vi "xijk_get_spectra.vi"(8 "error in":errorcluster, 10 "filepaths in":T2, 11 "spectra parameters in":T3={"Booleans"={"Notch filtering"=FALSE, "Unknown detector"=FALSE, "Dual band filters"=FALSE, "Dual emission by cubes"=FALSE, "FRET"=FALSE}, "Integers"={"Light source"=0, "Number of fluorophores"=0, "Wavelength of laser (nm) 1"=0, "Broadness of laser (nm) 1"=0.0, "Wavelength of laser (nm) 2"=0, "Broadness of laser (nm) 2"=0.0, "Template"=1}, "Doubles"={"Molar extinction 1"=1.0, "Molar extinction 2"=1.0, "Quantum efficiency 1"=1.0, "Quantum efficiency 2"=1.0}}) -> (0 "error out":errorcluster, 3 "spectra out":T1)   [LabVIEW 2010]
uses:
  Type Def/spectra_parameters.ctl
  Type Def/filepath.ctl
  Type Def/spectrum_table_control.ctl
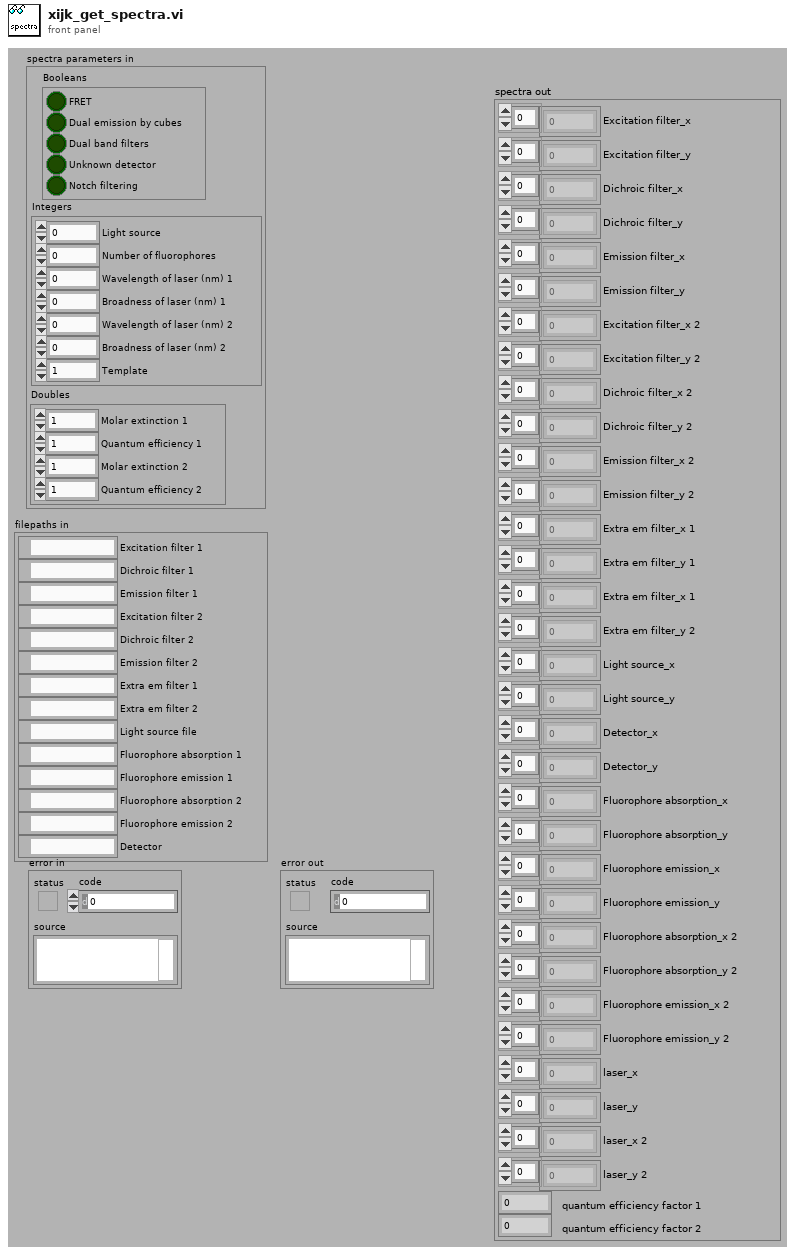
[diagram p1: front panel]
types:
  T1 = typedef "spectrum_table_control.ctl" = cluster{"Excitation filter_x":i16[], "Excitation filter_y":sgl[], "Dichroic filter_x":i16[], "Dichroic filter_y":sgl[], "Emission filter_x":i16[], "Emission filter_y":sgl[], "Excitation filter_x 2":i16[], "Excitation filter_y 2":sgl[], "Dichroic filter_x 2":i16[], "Dichroic filter_y 2":sgl[], "Emission filter_x 2":i16[], "Emission filter_y 2":sgl[], "Extra em filter_x 1":i16[], "Extra em filter_y 1":sgl[], "Extra em filter_x 1":i16[], "Extra em filter_y 2":sgl[], "Light source_x":i16[], "Light source_y":sgl[], "Detector_x":i16[], "Detector_y":sgl[], "Fluorophore absorption_x":i16[], "Fluorophore absorption_y":sgl[], "Fluorophore emission_x":i16[], "Fluorophore emission_y":sgl[], "Fluorophore absorption_x 2":i16[], "Fluorophore absorption_y 2":sgl[], "Fluorophore emission_x 2":i16[], "Fluorophore emission_y 2":sgl[], "laser_x":i16[], "laser_y":sgl[], "laser_x 2":i16[], "laser_y 2":sgl[], "quantum efficiency factor 1":sgl, "quantum efficiency factor 2":sgl}
  T2 = typedef "filepath.ctl" = cluster{"Excitation filter 1":path, "Dichroic filter 1":path, "Emission filter 1":path, "Excitation filter 2":path, "Dichroic filter 2":path, "Emission filter 2":path, "Extra em filter 1":path, "Extra em filter 2":path, "Light source file":path, "Fluorophore absorption 1":path, "Fluorophore emission 1":path, "Fluorophore absorption 2":path, "Fluorophore emission 2":path, "Detector":path}
  T3 = typedef "spectra_parameters.ctl" = cluster{"Booleans":cluster{"Notch filtering":bool, "Unknown detector":bool, "Dual band filters":bool, "Dual emission by cubes":bool, "FRET":bool}, "Integers":cluster{"Light source":u16, "Number of fluorophores":u16, "Wavelength of laser (nm) 1":u16, "Broadness of laser (nm) 1":sgl, "Wavelength of laser (nm) 2":u16, "Broadness of laser (nm) 2":sgl, "Template":u16}, "Doubles":cluster{"Molar extinction 1":sgl, "Molar extinction 2":sgl, "Quantum efficiency 1":sgl, "Quantum efficiency 2":sgl}}
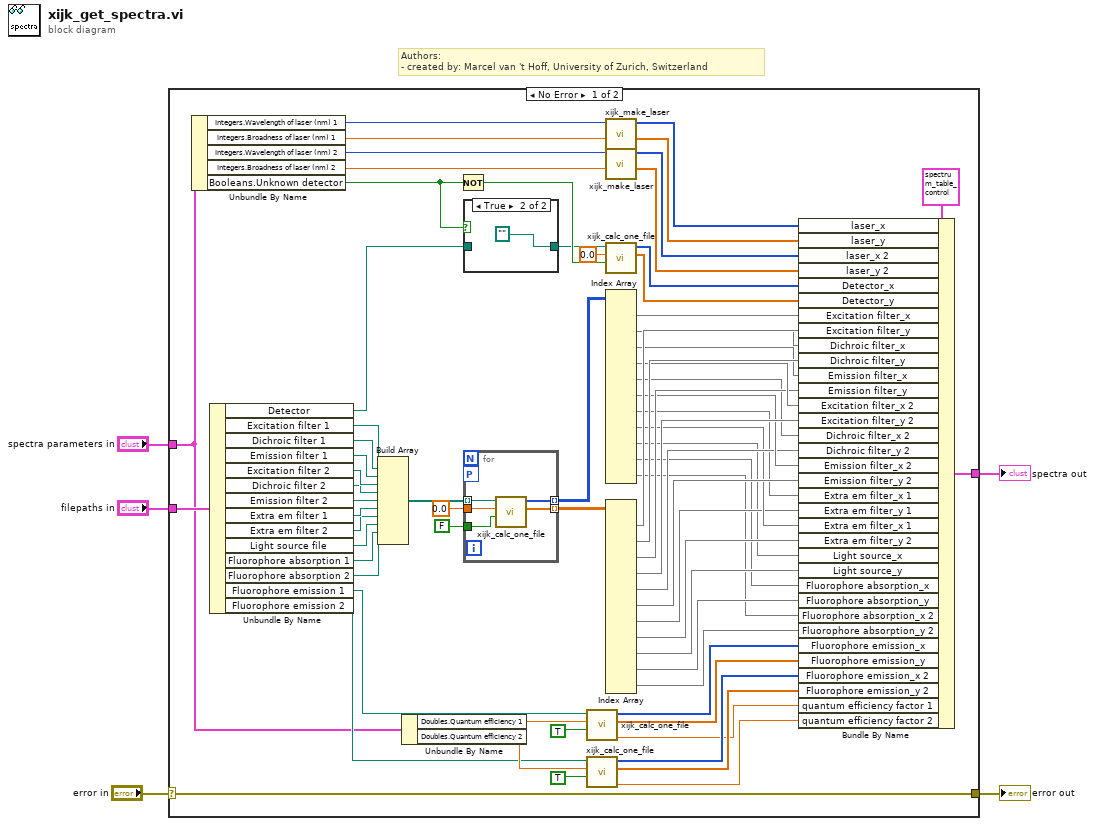
[diagram p0: block diagram]
diagram:
  # "Authors: \n- created by: Marcel van 't Hoff, University of Zurich, Switzerland"
  n1 = case shown="No Error" "error in" {
    selector: "error in" -> [w7 w83]
    tunnel: "filepaths in" -> [w75 _]
    tunnel: "spectra parameters in" -> [w50 _]
    tunnel: [w49 _] -> w3
    tunnel: [w7 w83] -> w1
    frame No Error {
      n2 = Unbundle By Name(w50) -> ("Integers.Wavelength of laser (nm) 1"=w56:u16, "Integers.Broadness of laser (nm) 1"=w55:sgl, "Integers.Wavelength of laser (nm) 2"=w54:u16, "Integers.Broadness of laser (nm) 2"=w53:sgl, "Booleans.Unknown detector"=w27:bool)
      n3 = Unbundle By Name(w75) -> ("Detector"=w28:path, "Excitation filter 1"=w74:path, "Dichroic filter 1"=w73:path, "Emission filter 1"=w72:path, "Excitation filter 2"=w71:path, "Dichroic filter 2"=w70:path, "Emission filter 2"=w69:path, "Extra em filter 1"=w68:path, "Extra em filter 2"=w64:path, "Light source file"=w67:path, "Fluorophore absorption 1"=w66:path, "Fluorophore absorption 2"=w65:path, "Fluorophore emission 1"=w52:path, "Fluorophore emission 2"=w51:path)
      n4 = Build Array(w74, w73, w72, w71, w70, w69, w68, w64, w67, w66, w65) -> (w63:path[])
      n5 = Unbundle By Name(w50) -> ("Doubles.Quantum efficiency 1"=w60:sgl, "Doubles.Quantum efficiency 2"=w57:sgl)
      n6 = Not(x=w27) -> (.not. x?=w26:bool)
      n7 = case shown="True" w27 {
        tunnel: w28 -> [w76 _]
        tunnel: [w76 path ""] -> w25
        frame False {
        }
        frame True {
        }
      }
      n8 = for {
        tunnel: w63 -> [w82] mode=indexing
        tunnel: [w81] -> w48 mode=indexing
        tunnel: [w80] -> w47 mode=indexing
        tunnel: sgl 0.0 ("quantum efficiency") -> [w79]
        tunnel: FALSE ("is_fluorophore") -> [w78]
        workers-P: _ -> [_]
        n9 = call "xijk_calc_one_file.vi"("is_fluorophore"=w78, "quantum efficiency"=w79, "input"=w82) -> ("y_out"=w80:sgl[], "x_out"=w81:i16[])  [unwired: 6 in, 1 out]
      }
      n10 = call "xijk_calc_one_file.vi"("is_fluorophore"=TRUE, "quantum efficiency"=w60, "input"=w52) -> ("quantum efficiency factor"=w9:sgl, "y_out"=w18:sgl[], "x_out"=w19:i16[])  [unwired: 6 in]
      n11 = call "xijk_calc_one_file.vi"("is_fluorophore"=TRUE, "quantum efficiency"=w57, "input"=w51) -> ("quantum efficiency factor"=w8:sgl, "y_out"=w16:sgl[], "x_out"=w17:i16[])  [unwired: 6 in]
      n12 = call "xijk_make_laser.vi"("Broadness of laser (nm)"=w55, "Wavelength of laser (nm)"=w56) -> ("laser_y"=w11:sgl[], "laser_x"=w10:i16[])  [unwired: 8 in]
      n13 = call "xijk_make_laser.vi"("Broadness of laser (nm)"=w53, "Wavelength of laser (nm)"=w54) -> ("laser_y"=w13:sgl[], "laser_x"=w12:i16[])  [unwired: 8 in]
      n14 = call "xijk_calc_one_file.vi"("is_fluorophore"=w26, "quantum efficiency"=sgl 0.0, "input"=w25) -> ("y_out"=w15:sgl[], "x_out"=w14:i16[])  [unwired: 6 in, 1 out]
      n15 = Index Array(array=w48) -> (element #1=w46:i16[], element #2=w44:i16[], element #3=w42:i16[], element #4=w41:i16[], element #5=w38:i16[], element #6=w37:i16[], element #7=w34:i16[], element #8=w33:i16[], element #9=w30:i16[], element #10=w23:i16[], element #11=w21:i16[])  [unwired: 22 in]
      n16 = Index Array(array=w47) -> (element #1=w45:sgl[], element #2=w43:sgl[], element #3=w40:sgl[], element #4=w39:sgl[], element #5=w36:sgl[], element #6=w35:sgl[], element #7=w32:sgl[], element #8=w31:sgl[], element #9=w29:sgl[], element #10=w22:sgl[], element #11=w20:sgl[])  [unwired: 22 in]
      n17 = Bundle By Name(cluster=T1 {"Excitation filter_x"=[], "Excitation filter_y"=[], "Dichroic filter_x"=[], "Dichroic filter_y"=[], "Emission filter_x"=[], "Emission filter_y"=[], "Excitation filter_x 2"=[], "Excitation filter_y 2"=[], "Dichroic filter_x 2"=[], "Dichroic filter_y 2"=[], "Emission filter_x 2"=[], "Emission filter_y 2"=[], "Extra em filter_x 1"=[], "Extra em filter_y 1"=[], "Extra em filter_x 1"=[], "Extra em filter_y 2"=[], "Light source_x"=[], "Light source_y"=[], "Detector_x"=[], "Detector_y"=[], "Fluorophore absorption_x"=[], "Fluorophore absorption_y"=[], "Fluorophore emission_x"=[], "Fluorophore emission_y"=[], "Fluorophore absorption_x 2"=[], "Fluorophore absorption_y 2"=[], "Fluorophore emission_x 2"=[], "Fluorophore emission_y 2"=[], "laser_x"=[], "laser_y"=[], "laser_x 2"=[], "laser_y 2"=[], "quantum efficiency factor 1"=0.0, "quantum efficiency factor 2"=0.0} ("spectra in"), "laser_x"=w10, "laser_y"=w11, "laser_x 2"=w12, "laser_y 2"=w13, "Detector_x"=w14, "Detector_y"=w15, "Excitation filter_x"=w46, "Excitation filter_y"=w45, "Dichroic filter_x"=w44, "Dichroic filter_y"=w43, "Emission filter_x"=w42, "Emission filter_y"=w40, "Excitation filter_x 2"=w41, "Excitation filter_y 2"=w39, "Dichroic filter_x 2"=w38, "Dichroic filter_y 2"=w36, "Emission filter_x 2"=w37, "Emission filter_y 2"=w35, "Extra em filter_x 1"=w34, "Extra em filter_y 1"=w32, "Extra em filter_x 1"=w33, "Extra em filter_y 2"=w31, "Light source_x"=w30, "Light source_y"=w29, "Fluorophore absorption_x"=w23, "Fluorophore absorption_y"=w22, "Fluorophore absorption_x 2"=w21, "Fluorophore absorption_y 2"=w20, "Fluorophore emission_x"=w19, "Fluorophore emission_y"=w18, "Fluorophore emission_x 2"=w17, "Fluorophore emission_y 2"=w16, "quantum efficiency factor 1"=w9, "quantum efficiency factor 2"=w8) -> (w49:T1)
    }
    frame Error {
    }
  }
  "spectra out" <- w3
  "error out" <- w1
